vi "DAQmx Create Channel (TEDS-AI-Voltage-Basic).vi"(0 "task in":refnum<k21>, 1 "maximum value":dbl=5.0 format="%0.2f", 2 "minimum value":dbl=-5.0 format="%0.2f", 3 "input terminal configuration":i32(ring)=-1 items=["default"=-1, "RSE"=10083, "NRSE"=10078, "Differential"=10106, "Pseudodifferential"=12529], 5 "physical channels":tag, 7 "name to assign":string, 9 "units":i32(ring)=12516 items=["From TEDS"=12516, "From Custom Scale"=10065], 11 "error in":errorcluster, 12 "custom scale name":tag) -> (4 "task out":refnum<k21>, 15 "error out":errorcluster)   [LabVIEW 2013]
doc: "Creates channel(s) to measure voltage. You must configure the physical channel(s) with TEDS information to use this VI. If the measurement requires the use of internal excitation or you need excitation to scale the voltage, use the TEDS AI Custom Voltage with Excitation instance of this VI."
uses:
  nilvaiu.dll
panel:
  # "input limits"
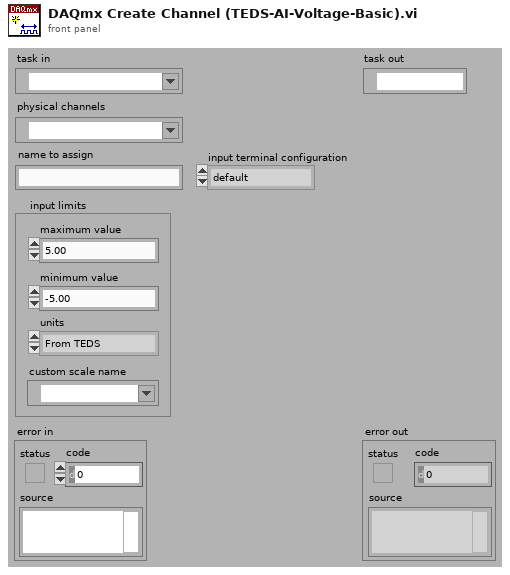
[diagram p1: front panel]
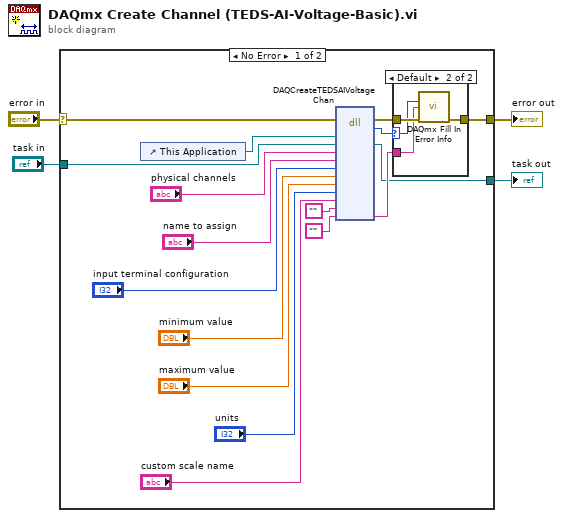
[diagram p0: block diagram]
diagram:
  n1 = case shown="No Error" "error in" {
    selector: "error in" -> [w8 w27]
    tunnel: "task in" -> [w10 w28]
    tunnel: [w9 w28] -> w3
    tunnel: [w7 w27] -> w1
    frame No Error {
      n2 = control-ref of="This Application"() -> (w17:refnum<vi>)
      n3 = dll-call lib="nilvaiu.*" fn="DAQCreateTEDSAIVoltageChan"(error in=w8, "lvAppRef"=w17, "refObjPtr"=w10, "physicalChannelName"="physical channels", "channelNameIn"="name to assign", "terminalConfig"="input terminal configuration", "minVal"="minimum value", "maxVal"="maximum value", "units"="units", "customScaleName"="custom scale name", "channelNamesOut"="", "extendedErrorInfo"="") -> (error out=w21:errorcluster, "return type"=w12:i32, "refObjPtr"=w9:refnum<k21>, "extendedErrorInfo"=w11:string)  [unwired: 11 in, 1 out]
      n4 = case shown="Default" w12 {
        selector: w12 -> [_ w24]
        tunnel: w21 -> [w22 w26]
        tunnel: [w22 w25] -> w7
        tunnel: w11 -> [_ w23]
        frame 0 {
        }
        frame Default {
          n5 = call "DAQmx Fill In Error Info.vi"("status code"=w24, "extended error info"=w23, "error in"=w26) -> ("error out"=w25:errorcluster)  [unwired: 1 in, 11 out]
        }
      }
    }
    frame Error {
    }
  }
  "task out" <- w3
  "error out" <- w1
